vi "FTW-Actor-Initialize.vi"(0 "FTW Actor Instance Type":refnum<class "FTW-ActorInstance.lvclass">, 5 "Initialization Job Sequence":string, 7 "Actor Instance Configuration":T1="{\n  \"Identity\": \"ActorName\",\n  \"InboxAddress\": \"tcp://127.0.0.1:*\",\n  \"PublisherAddress\": \"tcp://127.0.0.1:*\",\n  \"EnableInboxLogging\": true,\n  \"EnableJobLogging\": true\n}", 11 "error in":errorcluster) -> (4 "FTW Actor Instance":refnum<class "FTW-ActorInstance.lvclass">, 6 "Incoming Requests":refnum<event-registration>, 15 "error out":errorcluster)   [LabVIEW 2012, in "FTW-Actor.lvlib" / "FTW-ActorInstance.lvclass"]
uses:
  FTW-ActorInstance.lvclass
  Utility/FTW-Actor-Configuration.ctl
  Message/Request/FTW-Message-IncomingRequest.lvclass
  Utility/FTW-Actor-Address.ctl
  JobSequencer/FTW-JobSequencer.lvclass/FTW-JobSequencer.ctl
  EventLogger/FTW-Logger.lvclass
  FTW-ActorInstance.lvclass/FTW-ActorInstance.ctl
  Endpoint/FTW-Endpoint.lvclass
  <instcachedir>/0/FTW-JSON-ToLabVIEW_0E3E72F634BF4A9AB33E22111E055A26.lvgen/FTW-JSON-ToLabVIEW_0E3E72F634BF4A9AB33E22111E055A26_003.vi
  Core/JSON/FTW-JSON-RegexParse.vi
  Core/Regex/FTW-Regex.vi
  Core/JSON/FTW-JSON-RegexHeader.vi
  Core/Error/FTW-ERR-ThrowError.vi
  Core/Container/FTW-Container-Construct.vi
  Core/Container/FTW-Container-Load-JSON.vi
  Core/Container/FTW-Container-Destroy.vi
  JobSequencer/FTW-JobSequencer.lvclass
  Ether/FTW-Ether.lvclass
  FTW-Actor.lvlib
panel:
  # "Inputs"
  # "Outputs"
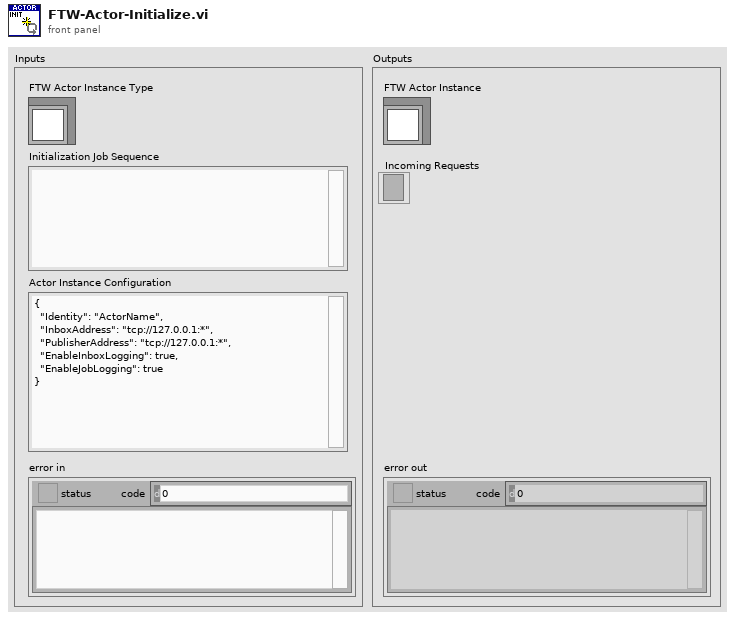
[diagram p1: front panel]
types:
  T1 = typedef "FTW-Actor.lvlib/FTW-Actor-Configuration.ctl" = string
  T2 = typedef "FTW-Actor.lvlib/FTW-Actor-Address.ctl" = string
  T3 = cluster{"Identity":string, "InboxAddress":T2, "PublisherAddress":T2, "LoggerAddress":T2, "LauncherAddress":T2, "EnableInboxLogging":bool, "EnableJobLogging":bool}
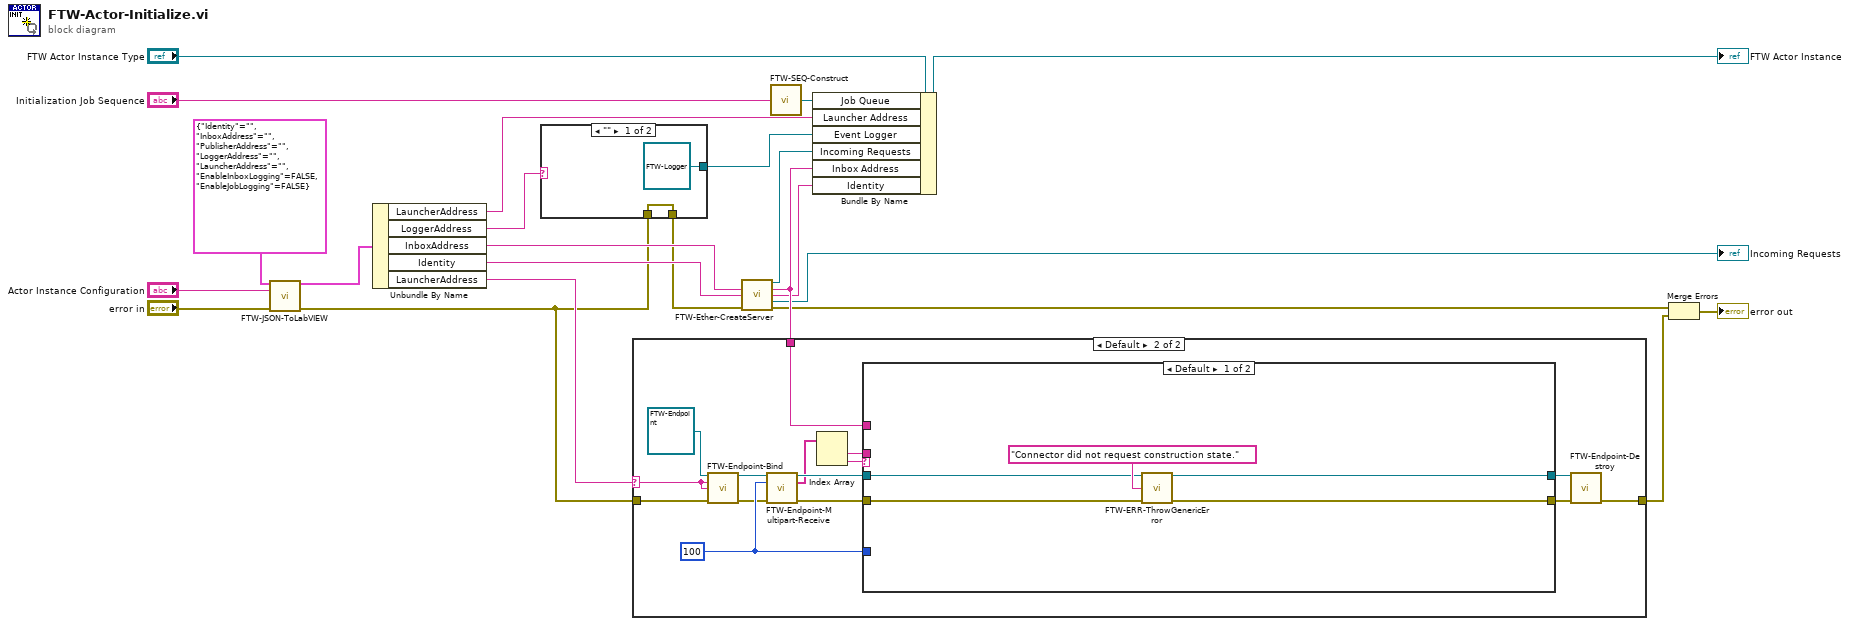
[diagram p0: block diagram]
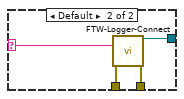
[diagram p2: hidden frame]
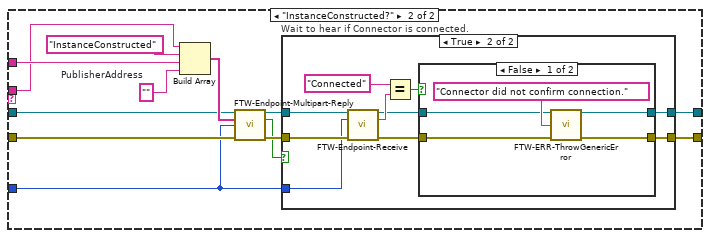
[diagram p4: hidden frame]
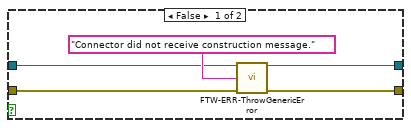
[diagram p5: hidden frame]
diagram:
  n1 = call-generic "FTW-JSON-ToLabVIEW.vi"("Type and Defaults"=T3 {"Identity"="", "InboxAddress"="", "PublisherAddress"="", "LoggerAddress"="", "LauncherAddress"="", "EnableInboxLogging"=FALSE, "EnableJobLogging"=FALSE}, "JSON String"="Actor Instance Configuration", "error in"="error in") -> ("Populated Values"=w14:T3, "error out"=w3:errorcluster)  [unwired: 11 in]
  n2 = Unbundle By Name(w14) -> ("LauncherAddress"=w8:T2, "LoggerAddress"=w1:T2, "InboxAddress"=w7:T2, "Identity"=w6:string, "LauncherAddress"=w12:T2)
  n3 = case shown="\"\"" w1 {
    selector: w1 -> [_ w26]
    tunnel: [refnum<class "FTW-Logger.lvclass"> refnum ("Event Logger Connection") w29] -> w4
    tunnel: w3 -> [w25 w28]
    tunnel: [w25 w27] -> w2
    frame "" {
    }
    frame Default {
      n4 = call "FTW-Logger-Connect.vi"("Logger Address"=w26, "error in"=w28) -> ("FTW Logger Connector"=w29:refnum<class "FTW-Logger.lvclass">, "error out"=w27:errorcluster)  [unwired: 12 in]
    }
  }
  n5 = call "FTW-Ether-CreateServer.vi"("Server Address"=w7, "Server Identity"=w6, "error in"=w2) -> ("Server Endpoint"=w18:refnum<class "FTW-Endpoint.lvclass">, "Actual Server Address"=w23:T2, "Actual Identity"=w13:string, "Incoming Requests"=→"Incoming Requests":refnum<event-registration>, "error out"=w11:errorcluster)  [unwired: 8 in]
  n6 = case shown="Default" w12 {
    selector: w12 -> [_ w31]
    tunnel: w3 -> [w30 w34]
    tunnel: w23 -> [_ w45]
    tunnel: [w30 w37] -> w10
    frame "" {
      # "There must not be a Launcher that wants to connect to this Instance."
    }
    frame Default {
      w43 = 100
      n7 = call-dynamic "FTW-Endpoint-Bind.vi"("FTW Endpoint"=refnum<class "FTW-Endpoint.lvclass"> refnum ("FTW Endpoint Type"), "Endpoint Address"=w31, "Requested Identity"=w31, "error in"=w34) -> ("FTW Endpoint out"=w33:refnum<class "FTW-Endpoint.lvclass">, "error out"=w32:errorcluster)  [unwired: 8 in, 2 out]
      n8 = call-dynamic "FTW-Endpoint-Multipart-Receive.vi"("FTW Endpoint"=w33, "Timeout"=w43, "error in"=w32) -> ("FTW Endpoint out"=w42:refnum<class "FTW-Endpoint.lvclass">, "Message Received"=w41:string[], "error out"=w44:errorcluster)  [unwired: 9 in, 1 out]
      n9 = Index Array(array=w41) -> (element #1=w39:string, element #2=w40:string)  [unwired: 2 in]
      n10 = case shown="Default" w40 {
        tunnel: w45 -> [_ w62]
        tunnel: w44 -> [w49 w58]
        tunnel: w43 -> [_ w53]
        tunnel: w42 -> [w46 w57]
        tunnel: w39 -> [_ w56]
        tunnel: [w48 w52] -> w36
        tunnel: [w46 w50] -> w38
        frame Default {
          n11 = call "FTW-ERR-ThrowGenericError.vi"("Error Message"="Connector did not request construction state.", "error in"=w49) -> ("error out"=w48:errorcluster)  [unwired: 13 in]
        }
        frame "InstanceConstructed?" {
          w60 = T2 ""  # PublisherAddress
          n12 = Build Array(w56, "InstanceConstructed", w62, w60) -> (w59:T2[])
          n13 = call-dynamic "FTW-Endpoint-Multipart-Reply.vi"("FTW Endpoint"=w57, "Multipart Message"=w59, "Timeout"=w53, "error in"=w58) -> ("FTW Endpoint out"=w55:refnum<class "FTW-Endpoint.lvclass">, "Timed out?"=w51:bool, "error out"=w54:errorcluster)  [unwired: 9 in]
          n14 = case "Wait to hear if Connector is connected." shown="True" w51 {
            tunnel: w55 -> [w63 w76]
            tunnel: w54 -> [w65 w75]
            tunnel: w53 -> [_ w74]
            tunnel: [w64 w67] -> w52
            tunnel: [w63 w68] -> w50
            frame False {
              n15 = call "FTW-ERR-ThrowGenericError.vi"("Error Message"="Connector did not receive construction message.", "error in"=w65) -> ("error out"=w64:errorcluster)  [unwired: 13 in]
            }
            frame True {
              n16 = call-dynamic "FTW-Endpoint-Receive.vi"("FTW Endpoint"=w76, "Timeout"=w74, "error in"=w75) -> ("FTW Endpoint out"=w70:refnum<class "FTW-Endpoint.lvclass">, "Response Header"=w72:string, "error out"=w69:errorcluster)  [unwired: 8 in, 2 out]
              n17 = Equal?(x="Connected" ("Message Header"), y=w72) -> (x = y?=w71:bool)
              n18 = case shown="False" w71 {
                tunnel: w70 -> [w78 w82]
                tunnel: w69 -> [w79 w81]
                tunnel: [w78 w82] -> w68
                tunnel: [w77 w81] -> w67
                frame False {
                  n19 = call "FTW-ERR-ThrowGenericError.vi"("Error Message"="Connector did not confirm connection.", "error in"=w79) -> ("error out"=w77:errorcluster)  [unwired: 13 in]
                }
                frame True {
                  # "All is good! This actor is duly initialized."
                }
              }
            }
          }
        }
      }
      n20 = call-dynamic "FTW-Endpoint-Destroy.vi"("FTW Endpoint"=w38, "error in"=w36) -> ("error out"=w37:errorcluster)  [unwired: 13 in]
    }
  }
  n21 = call "FTW-SEQ-Construct.vi"("Initial Sequence"="Initialization Job Sequence") -> ("FTW Job Sequencer"=w21:refnum<class "FTW-JobSequencer.lvclass">)
  n22 = Bundle By Name(cluster="FTW Actor Instance Type", "Job Queue"=w21, "Launcher Address"=w8, "Event Logger"=w4, "Incoming Requests"=w18, "Inbox Address"=w23, "Identity"=w13) -> (→"FTW Actor Instance":refnum<class "FTW-ActorInstance.lvclass">)
  n23 = Merge Errors(w11, w10) -> (→"error out":errorcluster)
